vi "Check Sim Controls.vi"(8 "error in (no error)":errorcluster, 11 "Simulation Controls":T2) -> (0 "error out":errorcluster, 3 "State":T1)   [LabVIEW 8.6]
doc: "This VI checks to see whether the pressure is below 50% or rain is present and sets the appropraite next state."
uses:
  Controls/State.ctl
panel:
  # "Rain"
  # "No Rain"
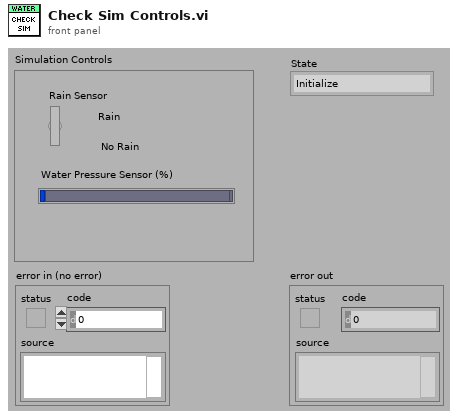
[diagram p1: front panel]
types:
  T1 = typedef "State.ctl" = enum16{"Initialize", "Idle", "Setup", "Start", "Running", "Low Water Pressure", "Rain", "Stop"}
  T2 = cluster{"Rain Sensor":bool, "Water Pressure Sensor (%)":dbl}
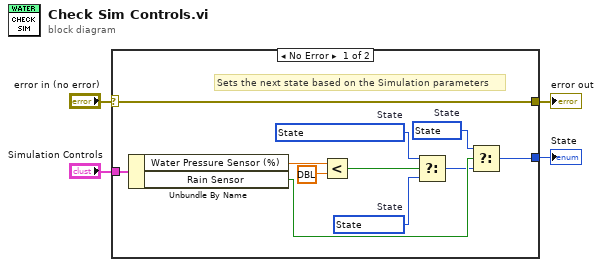
[diagram p0: block diagram]
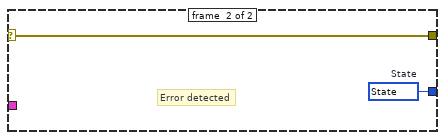
[diagram p2: hidden frame]
diagram:
  n1 = case shown="No Error" "error in (no error)" {
    selector: "error in (no error)" -> [w15 w17]
    tunnel: [w15 w17] -> w3
    tunnel: [w5 w16] -> w2
    tunnel: "Simulation Controls" -> [w14 _]
    frame #0 {
      w12 = T1 ?  # State
      w8 = T1 ?  # State
      w7 = T1 ?  # State
      # "Sets the next state based on the Simulation parameters"
      n2 = Unbundle By Name(w14) -> ("Water Pressure Sensor (%)"=w11:dbl, "Rain Sensor"=w13:bool)
      n3 = Less?(x=w11, y=dbl ?) -> (x < y?=w9:bool)
      n4 = Select(t=w8, s=w9, f=w7) -> (s? t:f=w6:T1)
      n5 = Select(t=w12, s=w13, f=w6) -> (s? t:f=w5:T1)
    }
    frame #1 {
      w16 = T1 ?  # State
      # "Error detected"
    }
  }
  "error out" <- w3
  "State" <- w2
